vi "Msg To.vi"() -> (3 "Teardown Msg out":refnum<class "Teardown Msg.lvclass">)   [LabVIEW 2021, in "Teardown.lvlib" / "Teardown Msg.lvclass"]
uses:
  Teardown Msg.lvclass
  Teardown Msg.lvclass/Teardown Msg.ctl
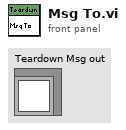
[diagram p1: front panel]
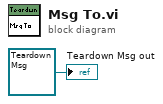
[diagram p0: block diagram]
diagram:
  "Teardown Msg out" <- refnum<class "Teardown Msg.lvclass"> refnum ("Destroy Msg in")
